vi "Configuration 2.0 Initialize.vi"(8 "error in (no error)":errorcluster, 10 "file version":T2, 11 "configuration json":string) -> (0 "error out":errorcluster, 3 "configuration 2.0":T1={"custom settings"=[], "plugins"=[{"core settings"={"component"="", "values"=[]}, "component settings"=[], "threads"=[{"core settings"={"component"="", "values"=[]}, "component settings"=[], "transfer groups"=[{"core settings"={"component"="Group", "values"=[]}, "component settings"=[], "transfers"=[{"core settings"={"component"="Transfer", "values"=[]}, "component settings"=[], "channels"=[{"core settings"={"component"="Channel", "values"=[]}, "component settings"=[]}]}]}]}]}]})   [LabVIEW 2021, in "DSF Core.lvlib" / "Configuration Session.lvclass"]
uses:
  Configuration Session.lvclass
  Typedefs/DSF Version Info.ctl
  DSF Core.lvlib
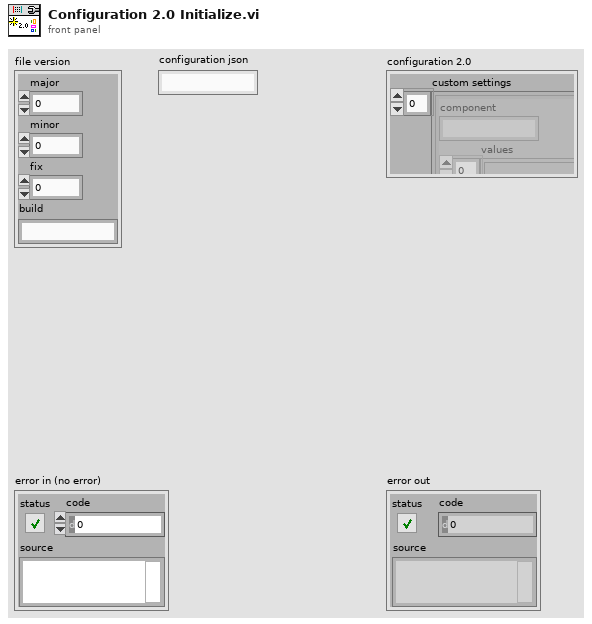
[diagram p1: front panel]
types:
  T1 = cluster{"custom settings":cluster{"component":string, "values":cluster{"key":string, "value":string}[]}[], "plugins":cluster{"core settings":cluster{"component":string, "values":cluster{"key":string, "value":string}[]}, "component settings":cluster{"component":string, "values":cluster{"key":string, "value":string}[]}[], "threads":cluster{"core settings":cluster{"component":string, "values":cluster{"key":string, "value":string}[]}, "component settings":cluster{"component":string, "values":cluster{"key":string, "value":string}[]}[], "transfer groups":cluster{"core settings":cluster{"component":string, "values":cluster{"key":string, "value":string}[]}, "component settings":cluster{"component":string, "values":cluster{"key":string, "value":string}[]}[], "transfers":cluster{"core settings":cluster{"component":string, "values":cluster{"key":string, "value":string}[]}, "component settings":cluster{"component":string, "values":cluster{"key":string, "value":string}[]}[], "channels":cluster{"core settings":cluster{"component":string, "values":cluster{"key":string, "value":string}[]}, "component settings":cluster{"component":string, "values":cluster{"key":string, "value":string}[]}[]}[]}[]}[]}[]}[]}
  T2 = typedef "DSF Core.lvlib/DSF Version Info.ctl" = cluster{"major":u32, "minor":u32, "fix":u32, "build":string}
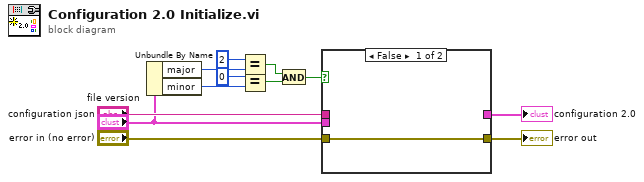
[diagram p0: block diagram]
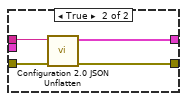
[diagram p2: hidden frame]
diagram:
  n1 = Unbundle By Name("file version") -> ("major"=w8:u32, "minor"=w11:u32)
  n2 = Equal?(x=u32 2, y=w8) -> (x = y?=w4:bool)
  n3 = Equal?(x=u32 0, y=w11) -> (x = y?=w5:bool)
  n4 = And(x=w4, y=w5) -> (x .and. y?=w3:bool)
  n5 = case shown="False" w3 {
    tunnel: "error in (no error)" -> [w13 w16]
    tunnel: "configuration json" -> [_ w17]
    tunnel: [_ w14] -> w10
    tunnel: [w13 w15] -> w9
    tunnel: "file version" -> [_ _]
    frame False {
    }
    frame True {
      n6 = call "Configuration 2.0 JSON Unflatten.vi"("error in (no error)"=w16, "dsf configuration json"=w17) -> ("error out"=w15:errorcluster, "configuration 2.0"=w14:T1)  [unwired: 8 in]
    }
  }
  "error out" <- w9
  "configuration 2.0" <- w10
